vi "3_AdvancedDemo_MHT3.vi"() -> ()   [LabVIEW 2017]
uses:
  Types/MH_InputChannel.ctl
  Types/MH_UIThread_Cmds.ctl
  Types/MH_UIThread_Data.ctl
  _lib/PQ/MultiHarp/MH_InitInfo.ctl
  Types/MH_DataProcThread_QData.ctl
  Types/MH_DataProcThread_QCmds.ctl
  Types/MH_VisThread_QData.ctl
  Types/MH_VisThread_QCmds.ctl
  Types/MH_VisThread_Data.ctl
  _lib/PQ/MultiHarp/MH_RefSource.ctl
  _lib/PQ/MultiHarp/MH_MeasMode.ctl
  <vilib>/Utility/error.llb/DialogType.ctl
  _lib/PQ/MultiHarp/mhlib_x86_x64_UIThread.llb/MH_DllPath_global.vi
  <vilib>/Utility/error.llb/Error Cluster From Error Code.vi
  _lib/PQ/MultiHarp/MH_LibVersion_global.vi
  <vilib>/ErrorRing/Error Ring.xnode
panel:
  in  "Settings":bool=TRUE
  in  "Run continuously":bool caption="Conti."
  in  "Start":bool
  in  "Scale":bool
  out "CountRates":i32[](graph)
  in  "HistoAcqTime":dbl=1.0 caption="Int.Time    s" min=0.1 max=360000.0 step=0.1
  in  "AcqTime":i32=360000000 caption="T3Acq.   ms" min=1 max=360000 step=1
  in  "Binning":i32(ring) caption="Resol.      ps" items=["80", "160", "320", "640", "1280", "2560", "5120", "10240", "20480", "40960", "81920", "163840", "327680", "655360", "1310720", "2621440", "5242880", "10485760", "20971520", "41943040", "83886080", "167772160", "335544320", "671088640", "1342177280", "2684354560"]
  in  "HistoOffset":i32 caption="Offset      ns" min=0 max=100000000 step=1
  out "DeltaT":dbl=3.2767475720388473 caption="Resol.     ms" format="%.2f"
  in  "BitShift":i32=15 min=0 max=32 step=1
  in  "OvlLevel":i32=65536 caption="Ovl.Level" min=1024 max=65536 step=1024
  in  "StopOvl.":bool=TRUE
  out "TTraceGraph":T1(graph)={0.0, "Resolution"=0.0032767475720388473, "Histogram"=[]}
  out "HistoGraph":cluster{dbl, "Resol":dbl, "Histos":u32[][]}(graph)={0.0, "Resol"=0.08, "Histos"=[]}
  in  "SyncEdge":i32(ring) caption="Edge" items=["falling", "rising"]
  in  "SyncDivider":i32(ring)=3 caption="Divider" items=["1", "2", "4", "8", "16"]
  in  "SyncOffset":i32 caption="Offset      ps" min=-99999 max=99999 step=1
  in  "SyncLevel":i32=-50 caption="Level      mV" min=-1200 max=1200 step=1
  in  "Channels":T2[](array[typedef])=[{"Name"="Inp.Chan 1", "Enable"=TRUE, "Offset"=0, "Level"=-50, "Edge"=0}, {"Name"="Inp.Chan 2", "Enable"=TRUE, "Offset"=0, "Level"=-50, "Edge"=0}, {"Name"="Inp.Chan 3", "Enable"=TRUE, "Offset"=0, "Level"=-50, "Edge"=0}, {"Name"="Inp.Chan 4", "Enable"=TRUE, "Offset"=0, "Level"=-50, "Edge"=0}, {"Name"="Inp.Chan 5", "Enable"=TRUE, "Offset"=0, "Level"=-50, "Edge"=0}, {"Name"="Inp.Chan 6", "Enable"=TRUE, "Offset"=0, "Level"=-50, "Edge"=0}, {"Name"="Inp.Chan 7", "Enable"=TRUE, "Offset"=0, "Level"=-50, "Edge"=0}, {"Name"="Inp.Chan 8", "Enable"=TRUE, "Offset"=0, "Level"=-50, "Edge"=0}] {"Edge" items=["falling", "rising"]; "Offset" min=-99999 max=99999 step=80; "Level" min=-1200 max=1200 step=1}
  out "SyncRate":string="Sync Rate: 10000160 cps\n"
  out "OverRun":bool caption="Overrun:"
  out "Status":string="Elements in Q: 0"
  # "Histogram"
  # "Time Trace"
  # "Sync"
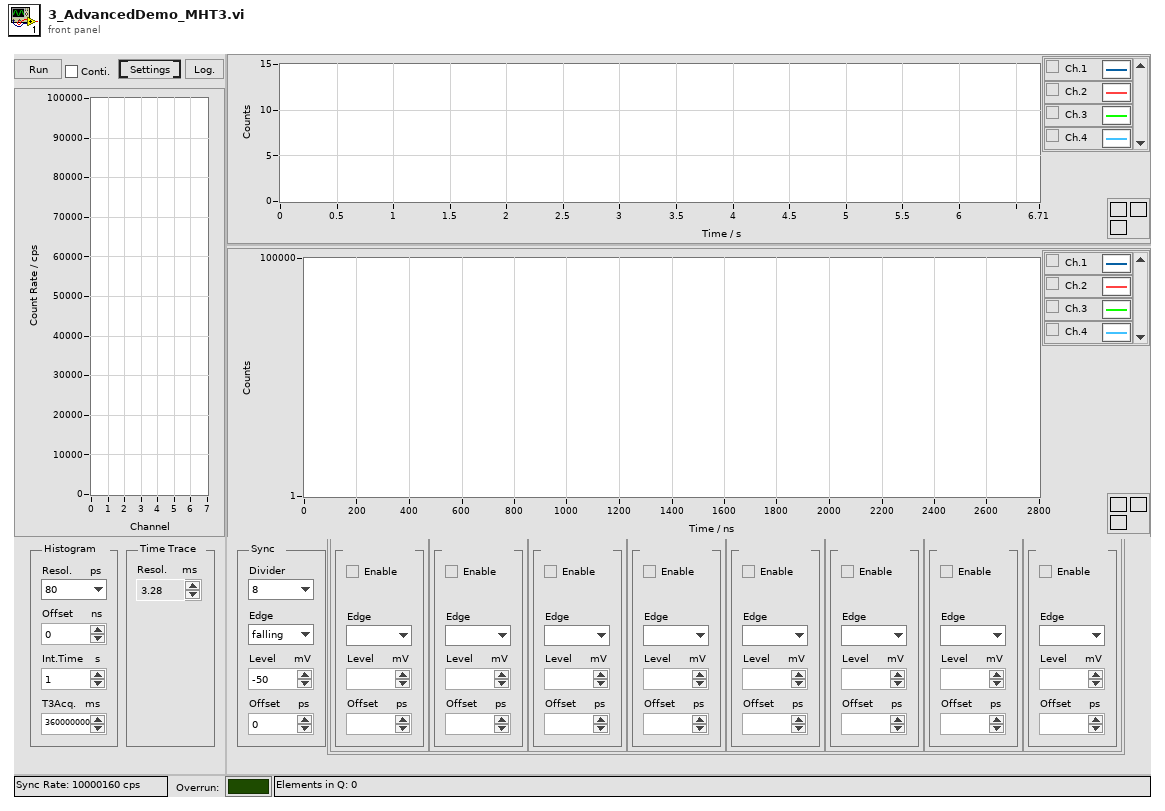
[diagram p1: front panel]
types:
  T1 = cluster{dbl, "Resolution":dbl, "Histogram":u32[][]}
  T2 = typedef "MH_InputChannel.ctl" = cluster{"Name":string, "Enable":bool, "Offset":i32, "Level":i32, "Edge":i32}
  T3 = typedef "MH_DataProcThread_QCmds.ctl" = enum16{"Exit", "Proc", "Init", "SetShift", "SetNumChannels", "SetHistAcqTime"}
  T4 = typedef "MH_VisThread_Data.ctl" = cluster{"Resol":dbl, "DeltaT":dbl, "NumChannels":i32}
  T5 = typedef "MH_VisThread_QData.ctl" = cluster{"Histos":u32[][], "Cmd":T6, "TimeTrace":u32[][], "Bin":i32, "Total bin":u64, "Status":string, "Resol":dbl, "DeltaT":dbl, "nChannels":i32}
  T6 = typedef "MH_VisThread_QCmds.ctl" = enum16{"_none_", "Resol", "nChannels", "DeltaT", "Histo", "TTrace", "Status"}
  T7 = typedef "MH_DataProcThread_QData.ctl" = cluster{"Cmd":T3, "nActual":i32, "Buffer":u32[], "TickCount":u32, "Param":i32}
  T8 = typedef "MH_UIThread_Data.ctl" = cluster{"Init Info":T9, "DevIdx":i32, "SyncDivider":i32, "SyncOffset":i32, "SyncLevel":i32, "Channels":T2[], "CurrentChannels":i32[], "AcqTime":i32, "Binning":i32, "HistoOffset":i32, "HistoLen":i32, "StopOvl.":bool, "OvlLevel":u32, "SyncEdge":i32, "StartMeas":bool, "HistoLength":i32, "Resolution":dbl, "Run cont.":bool, "Status":string, "SyncRate":i32, "BitShift":i32, "HistoAcqTime":dbl}
  T9 = typedef "MH_InitInfo.ctl" = cluster{"Library Version":string, "Serial No.":string, "Model":string, "Partnum":string, "Version":string, "features":i32, "nchannels":i32, "Base Resolution":dbl, "Bin Steps":i32}
  T10 = typedef "MH_UIThread_Cmds.ctl" = enum16{"Idle", "Init", "SetInpChanEnable", "SetInpChanOffset", "SetInpChanTrg", "SetSyncDivider", "SetSyncTrg", "SetSyncOffset", "SetBinning", "SetHistoOffset", "SetHistoLen", "SetStopOvl", "SetBitShift", "SetHistoAcqTime", "GetRates", "GetAllRates", "StartMeas", "StopMeas", "AbortMeas", "GetResolution", "GetHistos", "GetAllHistos", "ReadFiFo", "WriteStatus", "Resize", "EnableControls", "DisableControls", "Error", "Exit"}
  T11 = enum8{"Enabled", "Disabled", "Disabled and Grayed Out"}
  T12 = typedef "MH_MeasMode.ctl" = i32
  T13 = typedef "MH_RefSource.ctl" = enum16{"INTERNAL", "EXTERNAL_10MHZ", "WR_MASTER_GENERIC", "WR_SLAVE_GENERIC", "WR_GRANDM_GENERIC", "EXTN_GPS_PPS", "EXTN_GPS_PPS_UART", "WR_MASTER_MHARP", "WR_SLAVE_MHARP", "WR_GRANDM_MHARP"}
  T14 = typedef "DialogType.ctl" = u16
  T15 = cluster{"T0":dbl, "dt":dbl, "TimeTrace_out":u32[][]}
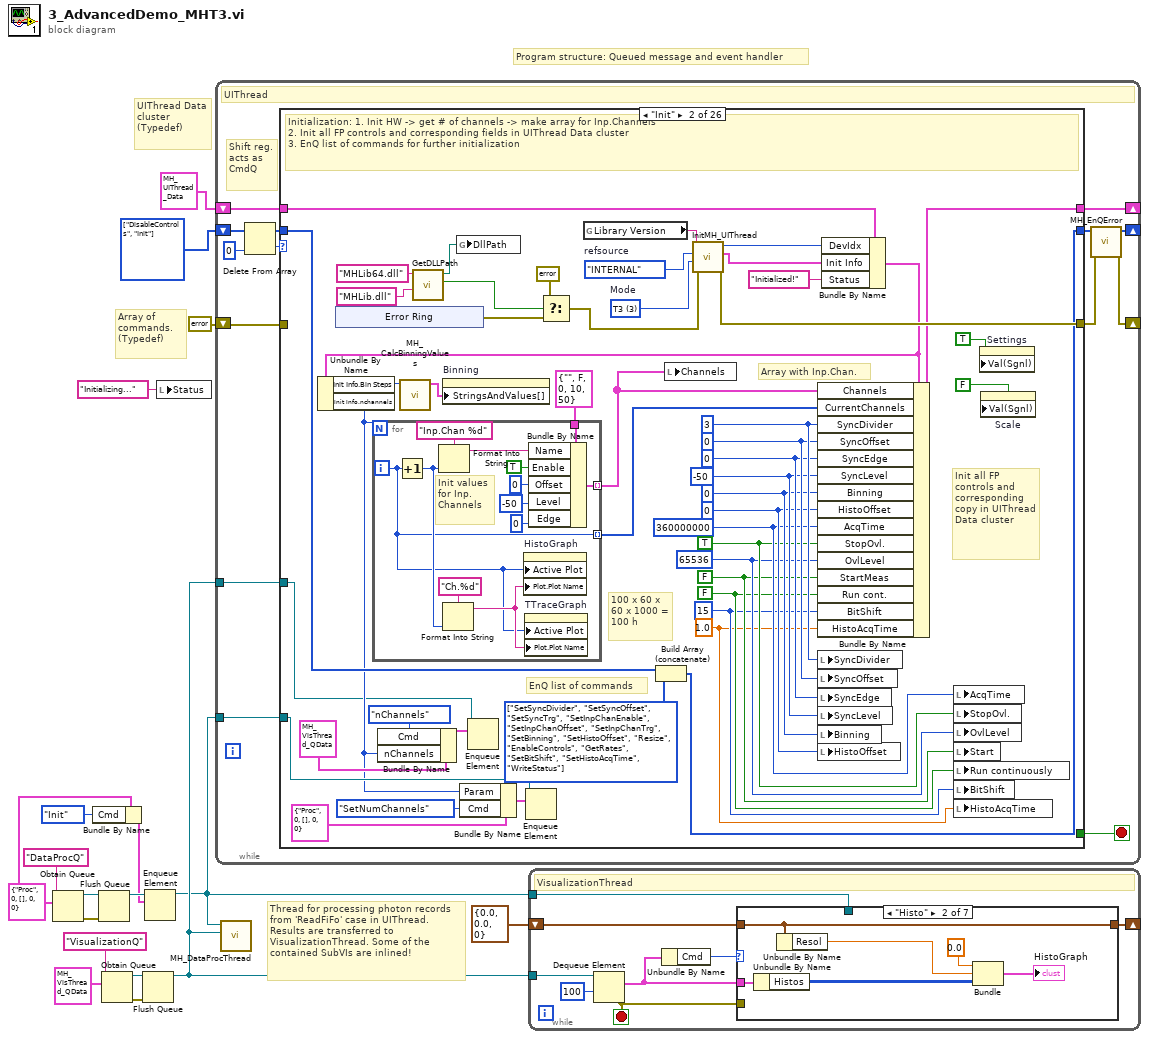
[diagram p0: block diagram]
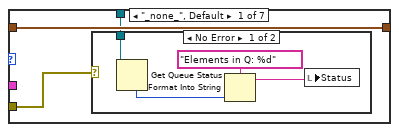
[diagram p2: hidden frame]
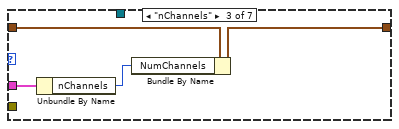
[diagram p4: hidden frame]
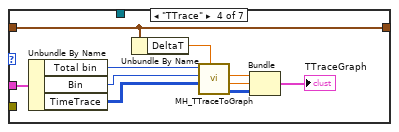
[diagram p5: hidden frame]
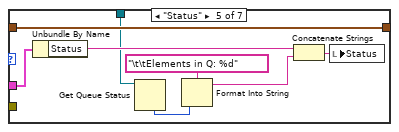
[diagram p6: hidden frame]
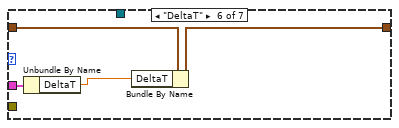
[diagram p7: hidden frame]
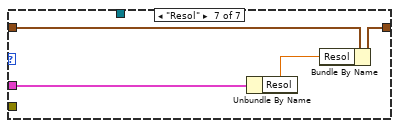
[diagram p8: hidden frame]
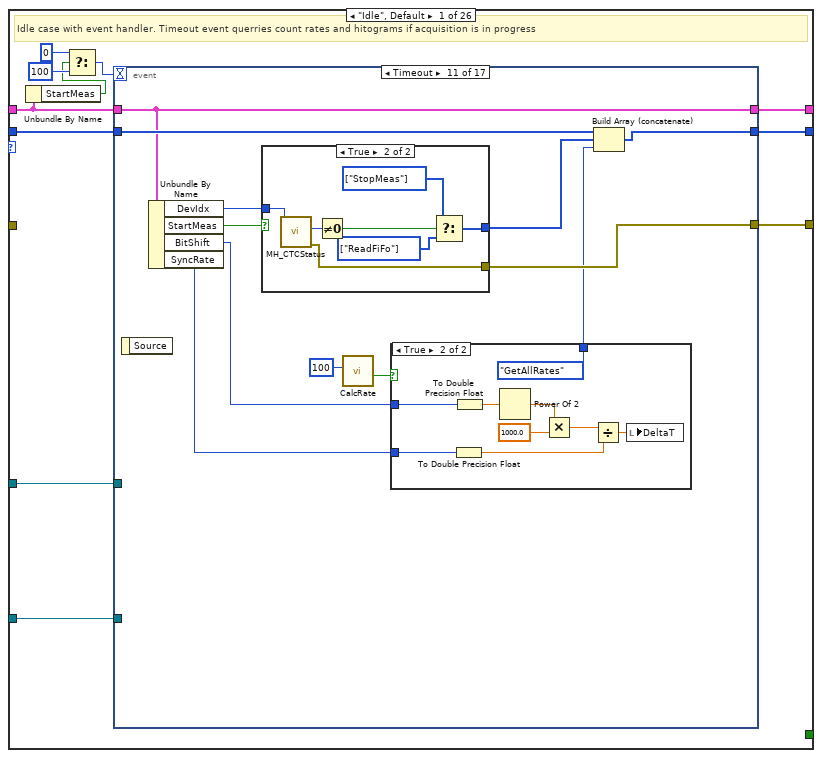
[diagram p9: hidden frame]
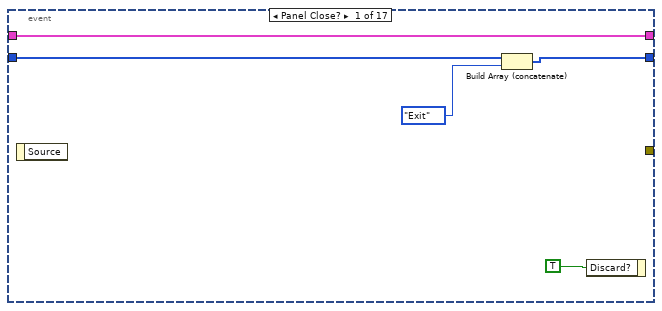
[diagram p10: hidden frame]
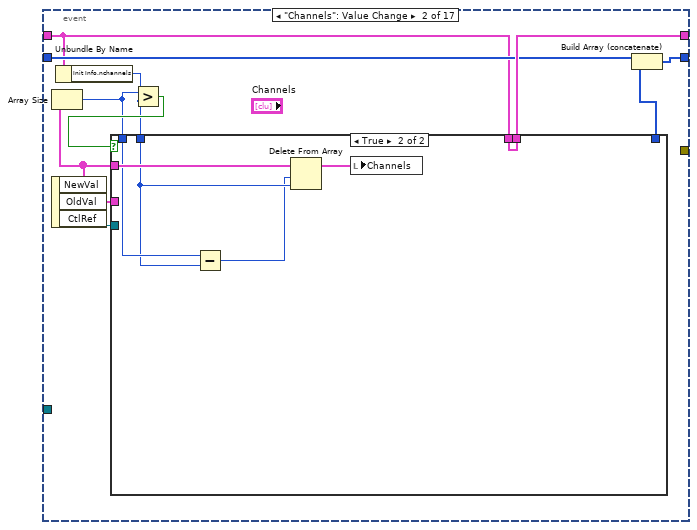
[diagram p11: hidden frame]
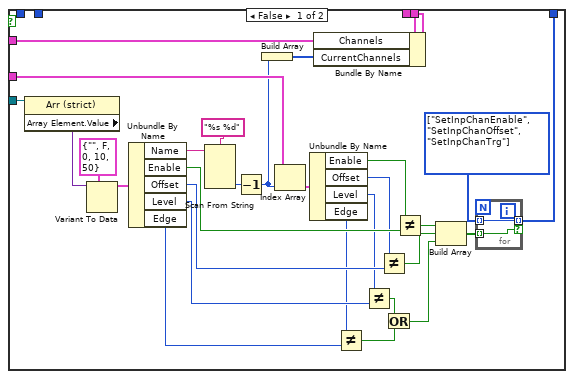
[diagram p12: hidden frame]
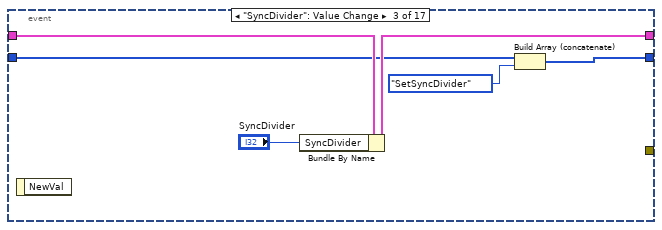
[diagram p13: hidden frame]
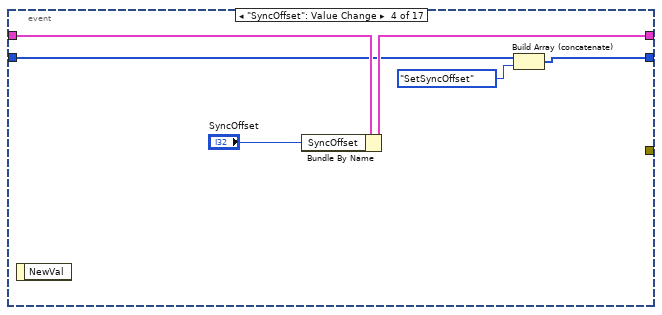
[diagram p14: hidden frame]
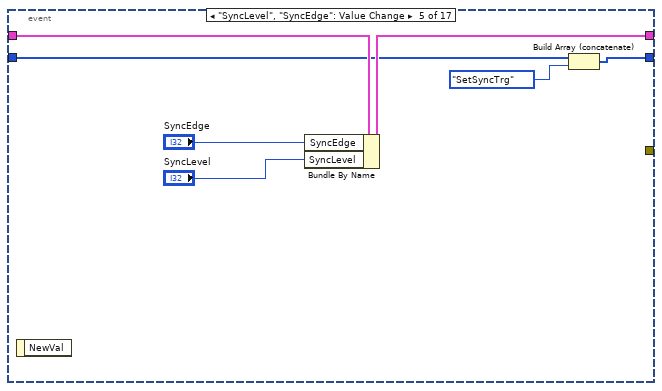
[diagram p15: hidden frame]
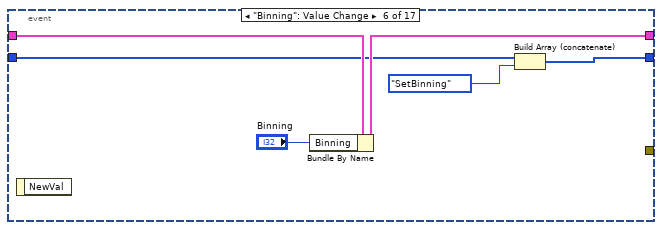
[diagram p16: hidden frame]
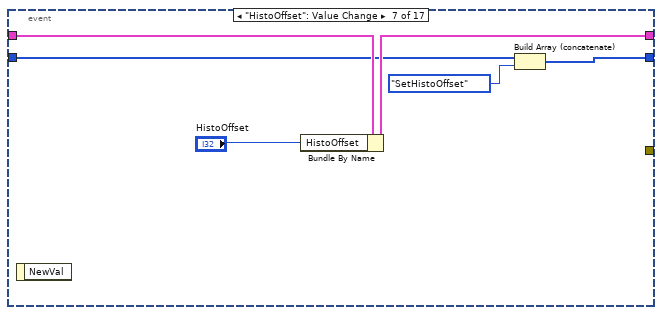
[diagram p17: hidden frame]
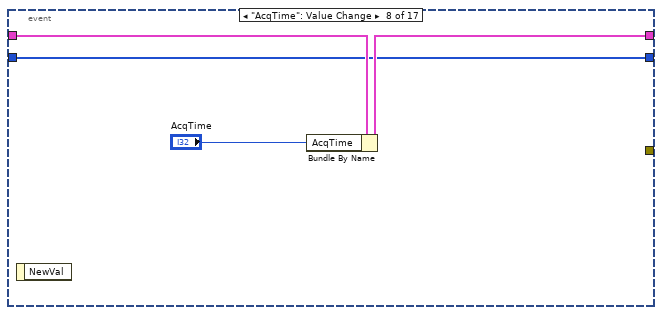
[diagram p18: hidden frame]
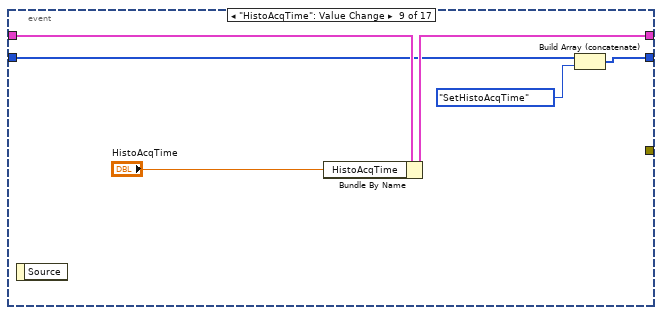
[diagram p19: hidden frame]
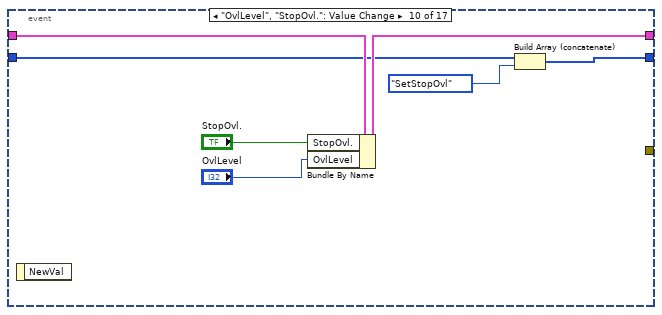
[diagram p20: hidden frame]
diagram:
  w4 = T7 {"Cmd"=enum."Proc", "nActual"=0, "Buffer"=[], "TickCount"=0, "Param"=0} ("MH_DataProcThread_QData")
  w17 = T10[] [enum."DisableControls", enum."Init"] items=["Idle", "Init", "SetInpChanEnable", "SetInpChanOffset", "SetInpChanTrg", "SetSyncDivider", "SetSyncTrg", "SetSyncOffset", "SetBinning", "SetHistoOffset", "SetHistoLen", "SetStopOvl", "SetBitShift", "SetHistoAcqTime", "GetRates", "GetAllRates", "StartMeas", "StopMeas", "AbortMeas", "GetResolution", "GetHistos", "GetAllHistos", "ReadFiFo", "WriteStatus", "Resize", "EnableControls", "DisableControls", "Error", "Exit"]
  # "Thread for processing photon records from 'ReadFiFo' case in UIThread. Results are transferred to VisualizationThread. Some of the contained SubVIs are inlined!"
  # "Array of commands.\n(Typedef)"
  # "Program structure: Queued message and event handler"
  # "UIThread Data cluster\n(Typedef)"
  n1 = Obtain Queue(name (unnamed)="DataProcQ", element data type=w4) -> (queue out=w14:refnum<queue>, error out=w13:errorcluster)  [unwired: 3 in, 1 out]
  n2 = Bundle By Name(cluster=w4, "Cmd"=MH_DataProcThread_QCmds."Init") -> (w2:T7)
  n3 = Flush Queue(queue=w14, error in (no error)=w13) -> (queue out=w5:refnum<queue>)  [unwired: 2 out]
  n4 = Obtain Queue(name (unnamed)="VisualizationQ", element data type=T5 {"Histos"=[], "Cmd"=enum."_none_", "TimeTrace"=[], "Bin"=0, "Total bin"=0, "Status"="", "Resol"=0.0, "DeltaT"=0.0, "nChannels"=0} ("MH_GUIThread_QData")) -> (queue out=w12:refnum<queue>, error out=w11:errorcluster)  [unwired: 3 in, 1 out]
  n5 = Flush Queue(queue=w12, error in (no error)=w11) -> (queue out=w7:refnum<queue>)  [unwired: 2 out]
  n6 = Enqueue Element(queue=w5, element=w2) -> (queue out=w1:refnum<queue>)  [unwired: 2 in, 2 out]
  n7 = local write "Status"("Initializing..." ("Status")) -> ()
  n8 = while {
    shift-right: [w21] -> _
    shift-left: w17 -> [w28]
    shift-right: [w31] -> _
    shift-left: T8 {"Init Info"={"Library Version"="", "Serial No."="", "Model"="", "Partnum"="", "Version"="", "features"=0, "nchannels"=0, "Base Resolution"=0.0, "Bin Steps"=0}, "DevIdx"=0, "SyncDivider"=1, "SyncOffset"=0, "SyncLevel"=50, "Channels"=[], "CurrentChannels"=[], "AcqTime"=1, "Binning"=1, "HistoOffset"=1, "HistoLen"=1024, "StopOvl."=FALSE, "OvlLevel"=1024, "SyncEdge"=10, "StartMeas"=FALSE, "HistoLength"=0, "Resolution"=0.0, "Run cont."=FALSE, "Status"="", "SyncRate"=0, "BitShift"=0, "HistoAcqTime"=0.0} -> [w30]
    shift-right: [w23] -> _
    shift-left: errorcluster {"status"=FALSE, "code"=0, "source"=""} ("error IO") -> [w29]
    tunnel: w1 -> [w20]
    tunnel: w7 -> [w19]
    stop <- w32 stop-if-true
    # "Shift reg.\nacts as\nCmdQ"
    # "UIThread"
    n9 = Delete From Array(array=w28, index=0) -> (deleted portion=w26:T10, array with subset deleted=w25:T10[])  [unwired: 1 in]
    n10 = case shown="\"Init\"" w26 {
      tunnel: [w43 w272 w301 w315 w329 w346 w355 w357 w364 w372 w379 w399 w411 w421 w433 w453 w459 w472 w489 w490 w516 w529 w536 w548 w554 w560] -> w22
      tunnel: [_ _ _ _ _ _ _ _ _ _ _ _ _ _ _ _ _ _ _ _ _ _ _ _ _ TRUE] -> w32
      tunnel: [w42 w253 w304 w318 w332 w348 w356 w361 w368 w373 w380 w384 w401 w415 w425 w457 w462 w474 w485 w500 w515 w517 w535 w547 w555 w563] -> w31
      tunnel: w30 -> [w39 w258 w304 w318 w332 w348 w356 w361 w368 w373 w380 w384 w401 w415 w426 w457 w463 w475 w486 w500 w515 w517 w535 w547 w555 w563]
      tunnel: [w40 w277 w302 w316 w330 w344 w354 w360 w367 w371 w378 _ _ w414 w432 w456 w465 w477 w487 w495 _ _ _ _ _ w561] -> w24
      tunnel: w29 -> [_ _ _ _ _ _ _ _ _ _ _ _ _ _ _ _ _ _ _ _ _ _ _ _ w556 _]
      tunnel: w25 -> [w41 w274 w301 w315 w329 w346 w355 w357 w363 w372 w379 w399 w411 w421 w433 w454 w460 w472 w489 w491 w516 w529 w536 w548 _ w560]
      tunnel: w20 -> [w34 w251 _ _ _ _ _ _ _ _ _ w385 w402 _ _ w450 _ _ _ w492 _ _ _ _ _ w559]
      tunnel: w19 -> [w33 w243 _ _ _ _ _ _ _ _ _ w386 _ _ _ _ _ _ w482 _ _ _ _ _ _ w558]
      frame "Idle", Default {
        # "Idle case with event handler. Timeout event querries count rates and hitograms if acquisition is in progress"
        n11 = Unbundle By Name(w39) -> ("StartMeas"=w37:bool)
        n12 = Select(t=0, s=w37, f=100) -> (s? t:f=w36:i32)
        n13 = event shown="[10] Timeout" {
          selector: _ -> [_ _ _ _ _ _ _ _ _ _ _ _ _ _ _ _ _]
          dyn-events: _ -> [_ _ _ _ _ _ _ _ _ _ _ _ _ _ _ _ _]
          timeout: w36 -> [_ _ _ _ _ _ _ _ _ _ _ _ _ _ _ _ _]
          tunnel: [w44 w54 w98 w104 w111 w118 w124 w129 w134 w141 w156 w174 w186 w204 w210 w218 w228] -> w43
          tunnel: [w47 w57 w102 w108 w115 w121 w127 w131 w137 w144 w155 w178 w185 w202 w209 w217 w231] -> w42
          tunnel: w39 -> [w47 w53 w103 w109 w116 w122 w128 w132 w138 w145 w155 w179 w183 w203 w209 w217 w231]
          tunnel: w41 -> [w46 w56 w100 w106 w113 w120 w126 w129 w135 w143 w157 w175 w187 w204 w210 w218 w229]
          tunnel: [_ _ _ _ _ _ _ _ _ _ w151 _ _ _ _ _ _] -> w40
          tunnel: w34 -> [_ _ _ _ _ _ _ _ _ _ _ _ _ _ _ _ _]
          tunnel: w33 -> [_ _ _ _ _ _ _ _ _ _ _ _ _ _ _ _ _]
          event Panel Close? {
            n14 = event-data() -> ()  [unwired: 1 in, 1 out]
            n15 = Build Array (concatenate)(w46, MH_UIThread_Cmds."Exit") -> (w44:T10[])
            n16 = event-data("Discard?"=TRUE) -> ()  [unwired: 1 in, 1 out]
          }
          event "Channels": Value Change {
            n17 = event-data() -> ("NewVal"=w52:T2[], "OldVal"=w58:T2[], "CtlRef"=w59:refnum<vi>)  [unwired: 1 in]
            n18 = Array Size(array=w52) -> (size(s)=w49:i32)
            n19 = Unbundle By Name(w53) -> ("Init Info.nchannels"=w50:i32)
            n20 = Greater?(x=w49, y=w50) -> (0:w51:bool)
            n21 = case shown="True" w51 {
              tunnel: w59 -> [w89 _]
              tunnel: w58 -> [w83 _]
              tunnel: [w66 w97] -> w57
              tunnel: [w64 _] -> w55
              tunnel: w53 -> [w61 w97]
              tunnel: w52 -> [w60 w96]
              tunnel: w50 -> [_ w94]
              tunnel: w49 -> [_ w95]
              frame False {
                w67 = T10[] [enum."SetInpChanEnable", enum."SetInpChanOffset", enum."SetInpChanTrg"] items=["Idle", "Init", "SetInpChanEnable", "SetInpChanOffset", "SetInpChanTrg", "SetSyncDivider", "SetSyncTrg", "SetSyncOffset", "SetBinning", "SetHistoOffset", "SetHistoLen", "SetStopOvl", "SetBitShift", "SetHistoAcqTime", "GetRates", "GetAllRates", "StartMeas", "StopMeas", "AbortMeas", "GetResolution", "GetHistos", "GetAllHistos", "ReadFiFo", "WriteStatus", "Resize", "EnableControls", "DisableControls", "Error", "Exit"]
                n22 = property class="Arr (strict)"(reference=w89) -> ("Array Element.Value"=w88:variant)  [unwired: 1 in, 2 out]
                n23 = Variant To Data(type=T2 {"Name"="", "Enable"=FALSE, "Offset"=0, "Level"=10, "Edge"=50} ("Channel"), Variant=w88) -> (data=w65:T2)  [unwired: 1 in, 1 out]
                n24 = Unbundle By Name(w65) -> ("Name"=w86:string, "Enable"=w80:bool, "Offset"=w78:i32, "Level"=w76:i32, "Edge"=w74:i32)
                n25 = Scan From String(format string="%s %d", input string=w86) -> (output 2=w84:i32)  [unwired: 5 in, 3 out]
                n26 = Decrement(x=w84) -> (x-1=w63:i32)
                n27 = Build Array(w63) -> (w62:i32[])
                n28 = Index Array(array=w83, index=w63) -> (element=w82:T2)
                n29 = Unbundle By Name(w82) -> ("Enable"=w81:bool, "Offset"=w79:i32, "Level"=w77:i32, "Edge"=w75:i32)
                n30 = Bundle By Name(cluster=w61, "Channels"=w60, "CurrentChannels"=w62) -> (w66:T8)
                n31 = Not Equal?(x=w75, y=w74) -> (x != y?=w69:bool)
                n32 = Not Equal?(x=w77, y=w76) -> (x != y?=w70:bool)
                n33 = Not Equal?(x=w79, y=w78) -> (x != y?=w72:bool)
                n34 = Or(x=w70, y=w69) -> (x .or. y?=w68:bool)
                n35 = Not Equal?(x=w81, y=w80) -> (x != y?=w73:bool)
                n36 = Build Array(w73, w72, w68) -> (w71:bool[])
                n37 = for {
                  tunnel: w71 -> [w90] mode=indexing
                  tunnel: w67 -> [w91] mode=indexing
                  tunnel: [w91] -> w64 mode=indexing if=w90
                }
              }
              frame True {
                n38 = Subtract(x=w95, y=w94) -> (x-y=w93:i32)
                n39 = Delete From Array(array=w96, length=w93, index=w94) -> (array with subset deleted=w92:T2[])  [unwired: 1 out]
                n40 = local write "Channels"(w92) -> ()
              }
            }
            n41 = Build Array (concatenate)(w56, w55) -> (w54:T10[])
          }
          event "SyncDivider": Value Change {
            n42 = event-data() -> ()  [unwired: 1 in, 1 out]
            n43 = Bundle By Name(cluster=w103, "SyncDivider"="SyncDivider") -> (w102:T8)
            n44 = Build Array (concatenate)(w100, MH_UIThread_Cmds."SetSyncDivider") -> (w98:T10[])
          }
          event "SyncOffset": Value Change {
            n45 = event-data() -> ()  [unwired: 1 in, 1 out]
            n46 = Bundle By Name(cluster=w109, "SyncOffset"="SyncOffset") -> (w108:T8)
            n47 = Build Array (concatenate)(w106, MH_UIThread_Cmds."SetSyncOffset") -> (w104:T10[])
          }
          event "SyncLevel", "SyncEdge": Value Change {
            n48 = event-data() -> ()  [unwired: 1 in, 1 out]
            n49 = Bundle By Name(cluster=w116, "SyncEdge"="SyncEdge", "SyncLevel"="SyncLevel") -> (w115:T8)
            n50 = Build Array (concatenate)(w113, MH_UIThread_Cmds."SetSyncTrg") -> (w111:T10[])
          }
          event "Binning": Value Change {
            n51 = event-data() -> ()  [unwired: 1 in, 1 out]
            n52 = Bundle By Name(cluster=w122, "Binning"="Binning") -> (w121:T8)
            n53 = Build Array (concatenate)(w120, MH_UIThread_Cmds."SetBinning") -> (w118:T10[])
          }
          event "HistoOffset": Value Change {
            n54 = event-data() -> ()  [unwired: 1 in, 1 out]
            n55 = Bundle By Name(cluster=w128, "HistoOffset"="HistoOffset") -> (w127:T8)
            n56 = Build Array (concatenate)(w126, MH_UIThread_Cmds."SetHistoOffset") -> (w124:T10[])
          }
          event "AcqTime": Value Change {
            n57 = event-data() -> ()  [unwired: 1 in, 1 out]
            n58 = Bundle By Name(cluster=w132, "AcqTime"="AcqTime") -> (w131:T8)
          }
          event "HistoAcqTime": Value Change {
            n59 = event-data() -> ()  [unwired: 1 in, 1 out]
            n60 = Bundle By Name(cluster=w138, "HistoAcqTime"="HistoAcqTime") -> (w137:T8)
            n61 = Build Array (concatenate)(w135, MH_UIThread_Cmds."SetHistoAcqTime") -> (w134:T10[])
          }
          event "OvlLevel", "StopOvl.": Value Change {
            n62 = event-data() -> ()  [unwired: 1 in, 1 out]
            n63 = Bundle By Name(cluster=w145, "StopOvl."="StopOvl.", "OvlLevel"="OvlLevel") -> (w144:T8)
            n64 = Build Array (concatenate)(w143, MH_UIThread_Cmds."SetStopOvl") -> (w141:T10[])
          }
          event Timeout {
            n65 = event-data() -> ()  [unwired: 1 in, 1 out]
            n66 = Unbundle By Name(w155) -> ("DevIdx"=w153:i32, "StartMeas"=w154:bool, "BitShift"=w150:i32, "SyncRate"=w149:i32)
            n67 = case shown="True" w154 {
              tunnel: w153 -> [_ w173]
              tunnel: [_ w171] -> w152
              tunnel: [_ w168] -> w151
              frame False {
              }
              frame True {
                w169 = T10[] [enum."ReadFiFo"] items=["Idle", "Init", "SetInpChanEnable", "SetInpChanOffset", "SetInpChanTrg", "SetSyncDivider", "SetSyncTrg", "SetSyncOffset", "SetBinning", "SetHistoOffset", "SetHistoLen", "SetStopOvl", "SetBitShift", "SetHistoAcqTime", "GetRates", "GetAllRates", "StartMeas", "StopMeas", "AbortMeas", "GetResolution", "GetHistos", "GetAllHistos", "ReadFiFo", "WriteStatus", "Resize", "EnableControls", "DisableControls", "Error", "Exit"]
                w170 = T10[] [enum."StopMeas"] items=["Idle", "Init", "SetInpChanEnable", "SetInpChanOffset", "SetInpChanTrg", "SetSyncDivider", "SetSyncTrg", "SetSyncOffset", "SetBinning", "SetHistoOffset", "SetHistoLen", "SetStopOvl", "SetBitShift", "SetHistoAcqTime", "GetRates", "GetAllRates", "StartMeas", "StopMeas", "AbortMeas", "GetResolution", "GetHistos", "GetAllHistos", "ReadFiFo", "WriteStatus", "Resize", "EnableControls", "DisableControls", "Error", "Exit"]
                n68 = call "MH_CTCStatus.vi"("devidx"=w173) -> ("error out"=w168:errorcluster, "ctcstatus"=w172:i32)  [unwired: 8 in, 1 out]
                n69 = Not Equal To 0?(x=w172) -> (x != 0?=w167:bool)
                n70 = Select(t=w170, s=w167, f=w169) -> (s? t:f=w171:T10[])
              }
            }
            n71 = call "CalcRate.vi"("Refresh(ms)"=u32 100) -> ("updated?"=w147:bool)  [unwired: 8 in, 2 out]
            n72 = case shown="True" w147 {
              tunnel: w150 -> [_ w160]
              tunnel: w149 -> [_ w159]
              tunnel: [_ MH_UIThread_Cmds."GetAllRates"] -> w148
              frame False {
              }
              frame True {
                n73 = To Double Precision Float(number=w159) -> (double precision float=w164:dbl)
                n74 = To Double Precision Float(number=w160) -> (double precision float=w165:dbl)
                n75 = Power Of 2(x=w165) -> (2^x=w163:dbl)
                n76 = Multiply(x=w163, y=1000.0) -> (x*y=w162:dbl)
                n77 = Divide(x=w162, y=w164) -> (x/y=w166:dbl)
                n78 = local write "DeltaT"(w166) -> ()
              }
            }
            n79 = Build Array (concatenate)(w157, w152, w148) -> (w156:T10[])
          }
          event "BitShift": Value Change {
            n80 = event-data() -> ()  [unwired: 1 in, 1 out]
            n81 = Bundle By Name(cluster=w179, "BitShift"="BitShift") -> (w178:T8)
            n82 = Build Array (concatenate)(w175, MH_UIThread_Cmds."SetBitShift") -> (w174:T10[])
          }
          event "Start": Value Change {
            n83 = event-data() -> ()  [unwired: 1 in, 1 out]
            n84 = Unbundle By Name(w183) -> ("SyncRate"=w182:i32)
            n85 = Greater Or Equal?(x=w182, y=10) -> (x >= y?=w180:bool)
            n86 = case shown="True" w180 {
              selector: w180 -> [w189 _]
              tunnel: w187 -> [w191 w200]
              tunnel: [w191 w198] -> w186
              tunnel: [w190 w197] -> w185
              tunnel: "Start" -> [_ w196]
              tunnel: w183 -> [w190 w192]
              frame False {
                n87 = local write "Start"(w189) -> ()
                n88 = One Button Dialog(message="SyncRate too low!!!" ("Status")) -> ()  [unwired: 1 in, 1 out]
              }
              frame True {
                w195 = T10[] [enum."SetBitShift", enum."SetHistoAcqTime", enum."StartMeas"] items=["Idle", "Init", "SetInpChanEnable", "SetInpChanOffset", "SetInpChanTrg", "SetSyncDivider", "SetSyncTrg", "SetSyncOffset", "SetBinning", "SetHistoOffset", "SetHistoLen", "SetStopOvl", "SetBitShift", "SetHistoAcqTime", "GetRates", "GetAllRates", "StartMeas", "StopMeas", "AbortMeas", "GetResolution", "GetHistos", "GetAllHistos", "ReadFiFo", "WriteStatus", "Resize", "EnableControls", "DisableControls", "Error", "Exit"]
                n89 = Bundle By Name(cluster=w192, "StartMeas"=w196) -> (w197:T8)
                n90 = Build Array(MH_UIThread_Cmds."AbortMeas") -> (w193:T10[])
                n91 = Select(t=w195, s=w196, f=w193) -> (s? t:f=w199:T10[])
                n92 = Build Array (concatenate)(w200, w199) -> (w198:T10[])
              }
            }
          }
          event "Run continuously": Value Change {
            n93 = event-data() -> ()  [unwired: 1 in, 1 out]
            n94 = Bundle By Name(cluster=w203, "Run cont."="Run continuously") -> (w202:T8)
          }
          event "Scale": Value Change {
            n95 = event-data() -> ()  [unwired: 1 in, 1 out]
            n96 = Select(t=u8 0 ("Y Scale.Mapping Mode"), s="Scale", f=u8 1 ("Y Scale.Mapping Mode")) -> (s? t:f=w205:u8)
            n97 = property on="HistoGraph" class="WFGraph (strict)"("YScale.Mapping Mode"=w205) -> ()  [unwired: 2 in, 2 out]
          }
          event "Settings": Value Change {
            n98 = event-data() -> ()  [unwired: 1 in, 1 out]
            n99 = property on="Splitter" class="Splitter"() -> ("Position"=w216:i32)  [unwired: 2 in, 2 out]
            n100 = Select(t=237 ("PosT"), s="Settings", f=0 ("PosF")) -> (s? t:f=w213:i32)
            n101 = Subtract(x=w216, y=w213) -> (x-y=w212:i32)
            n102 = while {
              shift-right: [w227] -> _
              shift-left: w212 -> [w220]
              i -> [w226]
              stop <- w223 stop-if-true
              n103 = property on="Splitter 4" class="Splitter"("Position"=w220) -> (error out=w219:errorcluster)  [unwired: 2 in, 1 out]
              n104 = Greater Or Equal?(x=w226, y=10) -> (x >= y?=w224:bool)
              n105 = Decrement(x=w220) -> (x-1=w227:i32)
              n106 = Unbundle(w219) -> ("status"=w222:bool)  [unwired: 2 out]
              n107 = Not(x=w222) -> (.not. x?=w221:bool)
              n108 = Or(x=w221, y=w224) -> (x .or. y?=w223:bool)
            }
          }
          event Panel Resize {
            n109 = event-data() -> ()  [unwired: 1 in, 1 out]
            n110 = Build Array (concatenate)(w229, MH_UIThread_Cmds."Resize") -> (w228:T10[])
          }
        }
      }
      frame "Init" {
        w232 = T12 3 items=["HIST"=0, "T2"=2, "T3"=3]  # Mode
        w234 = MH_RefSource."INTERNAL"  # refsource
        w241 = 1.0 ("HistoAcqTime")
        w242 = 15 ("Value (Signaling)")
        w260 = FALSE ("Run cont.")
        w262 = FALSE ("StartMeas")
        w263 = 65536 ("OvlLevel")
        w264 = TRUE ("StopOvl.")
        w265 = 360000000 ("AcqTime")
        w266 = 0 ("HistoOffset")
        w267 = 0 ("Binning")
        w268 = -50 ("SyncLevel")
        w269 = 0 ("SyncZeroX")
        w270 = 0 ("SyncOffset")
        w271 = 3 ("SyncDivider")
        w273 = T10[] [enum."SetSyncDivider", enum."SetSyncOffset", enum."SetSyncTrg", enum."SetInpChanEnable", enum."SetInpChanOffset", enum."SetInpChanTrg", enum."SetBinning", enum."SetHistoOffset", enum."Resize", enum."EnableControls", enum."GetRates", enum."SetBitShift", enum."SetHistoAcqTime", enum."WriteStatus"] items=["Idle", "Init", "SetInpChanEnable", "SetInpChanOffset", "SetInpChanTrg", "SetSyncDivider", "SetSyncTrg", "SetSyncOffset", "SetBinning", "SetHistoOffset", "SetHistoLen", "SetStopOvl", "SetBitShift", "SetHistoAcqTime", "GetRates", "GetAllRates", "StartMeas", "StopMeas", "AbortMeas", "GetResolution", "GetHistos", "GetAllHistos", "ReadFiFo", "WriteStatus", "Resize", "EnableControls", "DisableControls", "Error", "Exit"]
        # "100 x 60 x 60 x 1000 = 100 h"
        # "Init all FP controls and corresponding copy in UIThread Data cluster"
        # "EnQ list of commands"
        # "Array with Inp.Chan."
        # "Initialization: 1. Init HW -> get # of channels -> make array for Inp.Channels\n2. Init all FP controls and corresponding fields in UIThread Data cluster\n3. EnQ list of commands for further initialization"
        n111 = xnode "Error Ring"() -> ("error out"=w235:errorcluster)
        n112 = call "GetDLLPath.vi"("DllName_32bit"="MHLib.dll" ("name or relative path"), "DllName_64bit"="MHLib64.dll" ("name or relative path")) -> ("file exists?"=w237:bool, "DLLPath"=w238:path)  [unwired: 8 in]
        n113 = global write "MH_DllPath_global.vi" "DllPath"(w238) -> ()
        n114 = Select(t=errorcluster {"status"=FALSE, "code"=0, "source"=""} ("error IO"), s=w237, f=w235) -> (s? t:f=w254:errorcluster)
        n115 = global read "MH_LibVersion_global.vi" "Library Version"() -> (w233:string)
        n116 = Build Array (concatenate)(w274, w273) -> (w272:T10[])
        n117 = call "InitMH_UIThread.vi"("error in (no error)"=w254, "Mode"=w232, "refsource"=w234, "Library Version"=w233) -> ("error out"=w277:errorcluster, "Init Info"=w280:T9, "DevIdx"=w279:i32)  [unwired: 5 in]
        n118 = local write "SyncDivider"(w271) -> ()
        n119 = local write "SyncOffset"(w270) -> ()
        n120 = local write "SyncEdge"(w269) -> ()
        n121 = local write "SyncLevel"(w268) -> ()
        n122 = local write "Binning"(w267) -> ()
        n123 = local write "HistoOffset"(w266) -> ()
        n124 = Bundle By Name(cluster=w258, "DevIdx"=w279, "Init Info"=w280, "Status"="Initialized!") -> (w257:T8)
        n125 = Unbundle By Name(w257) -> ("Init Info.Bin Steps"=w256:i32, "Init Info.nchannels"=w244:i32)
        n126 = for {
          N: w244 -> [_]
          tunnel: T2 {"Name"="", "Enable"=FALSE, "Offset"=0, "Level"=10, "Edge"=50} ("Channel") -> [w297]
          tunnel: [w296] -> w276 mode=indexing
          tunnel: [w286] -> w275 mode=indexing
          i -> [w286]
          # "Init values for Inp. Channels"
          n127 = Increment(x=w286) -> (x+1=w289:i32)
          n128 = Format Into String(format string="Inp.Chan %d", w289) -> (resulting string=w294:string)  [unwired: 2 in, 1 out]
          n129 = Format Into String(format string="Ch.%d", w289) -> (resulting string=w287:string)  [unwired: 2 in, 1 out]
          n130 = property on="HistoGraph" class="WFGraph (strict)"("Active Plot"=w286, "Plot.Plot Name"=w287) -> ()  [unwired: 2 in, 2 out]
          n131 = property on="TTraceGraph" class="WFGraph (strict)"("Active Plot"=w286, "Plot.Plot Name"=w287) -> ()  [unwired: 2 in, 2 out]
          n132 = Bundle By Name(cluster=w297, "Name"=w294, "Enable"=TRUE, "Offset"=0, "Level"=-50 ("CFDZeroX"), "Edge"=0 ("CFDLevel")) -> (w296:T2)
        }
        n133 = Bundle By Name(cluster=T5 {"Histos"=[], "Cmd"=enum."_none_", "TimeTrace"=[], "Bin"=0, "Total bin"=0, "Status"="", "Resol"=0.0, "DeltaT"=0.0, "nChannels"=0} ("MH_GUIThread_QData"), "Cmd"=MH_VisThread_QCmds."nChannels", "nChannels"=w244) -> (w246:T5)
        n134 = call "MH_CalcBinningValues.vi"("Bin Steps"=w256) -> ("BinningValues"=w261:cluster{"String":string, "Value":i32}[])  [unwired: 10 in]
        n135 = property on="Binning" class="Ring (strict)"("StringsAndValues[]"=w261) -> ()  [unwired: 2 in, 2 out]
        n136 = Bundle By Name(cluster=T7 {"Cmd"=enum."Proc", "nActual"=0, "Buffer"=[], "TickCount"=0, "Param"=0} ("MH_DataProcThread_QData"), "Param"=w244, "Cmd"=MH_DataProcThread_QCmds."SetNumChannels") -> (w250:T7)
        n137 = Enqueue Element(queue=w243, element=w246) -> ()  [unwired: 2 in, 3 out]
        n138 = Enqueue Element(queue=w251, element=w250) -> ()  [unwired: 2 in, 3 out]
        n139 = local write "Channels"(w276) -> ()
        n140 = Bundle By Name(cluster=w257, "Channels"=w276, "CurrentChannels"=w275, "SyncDivider"=w271, "SyncOffset"=w270, "SyncEdge"=w269, "SyncLevel"=w268, "Binning"=w267, "HistoOffset"=w266, "AcqTime"=w265, "StopOvl."=w264, "OvlLevel"=w263, "StartMeas"=w262, "Run cont."=w260, "BitShift"=w242, "HistoAcqTime"=w241) -> (w253:T8)
        n141 = local write "AcqTime"(w265) -> ()
        n142 = local write "StopOvl."(w264) -> ()
        n143 = local write "OvlLevel"(w263) -> ()
        n144 = local write "Start"(w262) -> ()
        n145 = local write "Run continuously"(w260) -> ()
        n146 = local write "BitShift"(w242) -> ()
        n147 = local write "HistoAcqTime"(w241) -> ()
        n148 = property on="Settings" class="Bool (strict)"("Val(Sgnl)"=TRUE ("Value (Signaling)")) -> ()  [unwired: 2 in, 2 out]
        n149 = property on="Scale" class="Bool (strict)"("Val(Sgnl)"=FALSE ("Value (Signaling)")) -> ()  [unwired: 2 in, 2 out]
      }
      frame "SetInpChanEnable" {
        n150 = Unbundle By Name(w304) -> ("DevIdx"=w303:i32, "Channels"=w298:T2[], "CurrentChannels"=w299:i32[])
        n151 = for {
          tunnel: w303 -> [w311]
          shift-right: [w310] -> w302
          shift-left: errorcluster {"status"=FALSE, "code"=0, "source"=""} ("error out") -> [w309]
          tunnel: w299 -> [w305] mode=indexing
          tunnel: w298 -> [w308]
          n152 = Index Array(array=w308, index=w305) -> (element=w307:T2)
          n153 = Unbundle By Name(w307) -> ("Enable"=w306:bool)
          n154 = call "MH_SetInputChannelEnable.vi"("error in (no error)"=w309, "enable"=w306, "channel"=w305, "devidx"=w311) -> ("error out"=w310:errorcluster)  [unwired: 6 in, 1 out]
        }
      }
      frame "SetInpChanOffset" {
        n155 = Unbundle By Name(w318) -> ("DevIdx"=w317:i32, "Channels"=w312:T2[], "CurrentChannels"=w313:i32[])
        n156 = for {
          tunnel: w317 -> [w323]
          shift-right: [w320] -> w316
          shift-left: errorcluster {"status"=FALSE, "code"=0, "source"=""} ("error out") -> [w321]
          tunnel: w313 -> [w322] mode=indexing
          tunnel: w312 -> [w325]
          n157 = Index Array(array=w325, index=w322) -> (element=w324:T2)
          n158 = Unbundle By Name(w324) -> ("Offset"=w319:i32)
          n159 = call "MH_SetInputChannelOffset.vi"("error in (no error)"=w321, "Offset"=w319, "channel"=w322, "devidx"=w323) -> ("error out"=w320:errorcluster)  [unwired: 6 in, 1 out]
        }
      }
      frame "SetInpChanTrg" {
        n160 = Unbundle By Name(w332) -> ("DevIdx"=w331:i32, "Channels"=w326:T2[], "CurrentChannels"=w327:i32[])
        n161 = for {
          tunnel: w331 -> [w335]
          shift-right: [w337] -> w330
          shift-left: errorcluster {"status"=FALSE, "code"=0, "source"=""} ("error out") -> [w338]
          tunnel: w327 -> [w336] mode=indexing
          tunnel: w326 -> [w340]
          n162 = Index Array(array=w340, index=w336) -> (element=w339:T2)
          n163 = Unbundle By Name(w339) -> ("Level"=w334:i32, "Edge"=w333:i32)
          n164 = call "MH_SetInputEdgeTrg.vi"("channel"=w336, "error in (no error)"=w338, "edge"=w333, "level"=w334, "devidx"=w335) -> ("error out"=w337:errorcluster)  [unwired: 5 in, 1 out]
        }
      }
      frame "SetSyncDivider" {
        n165 = Unbundle By Name(w348) -> ("DevIdx"=w347:i32, "SyncDivider"=w343:i32)
        n166 = Power Of 2(x=w343) -> (2^x=w342:dbl)
        n167 = To Long Integer(number=w342) -> (32bit integer=w341:i32)
        n168 = call "MH_SetSyncDiv.vi"("SyncDivider"=w341, "devidx"=w347) -> ("error out"=w345:errorcluster)  [unwired: 8 in, 1 out]
        n169 = flat-sequence {
          tunnel: w345 -> [w349]
          tunnel: [w349] -> w344
          frame #0 {
            n170 = Wait (ms)(milliseconds to wait=u32 100) -> ()  [unwired: 1 out]
          }
        }
      }
      frame "SetSyncTrg" {
        n171 = Unbundle By Name(w356) -> ("DevIdx"=w353:i32, "SyncLevel"=w351:i32, "SyncEdge"=w352:i32)
        n172 = call "MH_SetSyncEdgeTrg.vi"("edge"=w352, "level"=w351, "devidx"=w353) -> ("error out"=w354:errorcluster)  [unwired: 7 in, 1 out]
      }
      frame "SetSyncOffset" {
        n173 = Unbundle By Name(w361) -> ("DevIdx"=w359:i32, "SyncOffset"=w358:i32)
        n174 = call "MH_SetSyncChannelOffset.vi"("Offset"=w358, "devidx"=w359) -> ("error out"=w360:errorcluster)  [unwired: 8 in, 1 out]
      }
      frame "SetBinning" {
        # "When binning is changed the new resolution is querried"
        n175 = Unbundle By Name(w368) -> ("DevIdx"=w366:i32, "Binning"=w365:i32)
        n176 = call "MH_SetBinning.vi"("Binning"=w365, "devidx"=w366) -> ("error out"=w367:errorcluster)  [unwired: 8 in, 1 out]
        n177 = Build Array (concatenate)(MH_UIThread_Cmds."GetResolution", w363) -> (w364:T10[])
      }
      frame "SetHistoOffset" {
        n178 = Unbundle By Name(w373) -> ("DevIdx"=w370:i32, "HistoOffset"=w369:i32)
        n179 = call "MH_SetOffset.vi"("Offset"=w369, "devidx"=w370) -> ("error out"=w371:errorcluster)  [unwired: 8 in, 1 out]
      }
      frame "SetStopOvl" {
        n180 = Unbundle By Name(w380) -> ("DevIdx"=w377:i32, "StopOvl."=w376:bool, "OvlLevel"=w375:u32)
        n181 = To Unsigned Long Integer(number=w375) -> (unsigned 32bit integer=w374:u32)
        n182 = call "MH_SetStopOverflow.vi"("stopcount"=w374, "StopOnOverflow"=w376, "devidx"=w377) -> ("error out"=w378:errorcluster)  [unwired: 7 in, 1 out]
      }
      frame "SetBitShift" {
        n183 = Unbundle By Name(w384) -> ("BitShift"=w382:i32, "SyncRate"=w383:i32)
        n184 = Negate(x=w382) -> (-x=w392:i32)
        n185 = Bundle By Name(cluster=T7 {"Cmd"=enum."Proc", "nActual"=0, "Buffer"=[], "TickCount"=0, "Param"=0} ("MH_DataProcThread_QData"), "Param"=w392, "Cmd"=MH_DataProcThread_QCmds."SetShift") -> (w398:T7)
        n186 = To Double Precision Float(number=w382) -> (double precision float=w397:dbl)
        n187 = To Double Precision Float(number=w383) -> (double precision float=w396:dbl)
        n188 = Power Of 2(x=w397) -> (2^x=w395:dbl)
        n189 = Enqueue Element(queue=w385, element=w398) -> ()  [unwired: 2 in, 3 out]
        n190 = Multiply(x=w395, y=1000.0) -> (x*y=w394:dbl)
        n191 = Divide(x=w394, y=w396) -> (x/y=w381:dbl)
        "DeltaT" <- w381
        n192 = Bundle By Name(cluster=T5 {"Histos"=[], "Cmd"=enum."_none_", "TimeTrace"=[], "Bin"=0, "Total bin"=0, "Status"="", "Resol"=0.0, "DeltaT"=0.0, "nChannels"=0} ("MH_GUIThread_QData"), "DeltaT"=w381, "Cmd"=MH_VisThread_QCmds."DeltaT") -> (w393:T5)
        n193 = Enqueue Element(queue=w386, element=w393) -> ()  [unwired: 2 in, 3 out]
      }
      frame "SetHistoAcqTime" {
        n194 = Unbundle By Name(w401) -> ("SyncRate"=w407:i32, "HistoAcqTime"=w400:dbl)
        n195 = To Double Precision Float(number=w407) -> (double precision float=w410:dbl)
        n196 = Multiply(x=w410, y=w400) -> (x*y=w409:dbl)
        n197 = Round To Nearest(number=w409) -> (nearest integer value=w408:dbl)
        n198 = To Long Integer(number=w408) -> (32bit integer=w406:i32)
        n199 = Bundle By Name(cluster=T7 {"Cmd"=enum."Proc", "nActual"=0, "Buffer"=[], "TickCount"=0, "Param"=0} ("MH_DataProcThread_QData"), "Param"=w406, "Cmd"=MH_DataProcThread_QCmds."SetHistAcqTime") -> (w405:T7)
        n200 = Enqueue Element(queue=w402, element=w405) -> ()  [unwired: 2 in, 3 out]
      }
      frame "GetAllRates" {
        # "An alternative to GetRates"
        n201 = Unbundle By Name(w415) -> ("DevIdx"=w417:i32, "Init Info.nchannels"=w420:i32)
        n202 = call "MH_AllocateCntRateBuffer.vi"("NumChan"=w420) -> ("Buffer"=w419:i32[])  [unwired: 10 in]
        n203 = call "MH_GetAllCountRates.vi"("cntrates_buf"=w419, "devidx"=w417) -> ("error out"=w414:errorcluster, "cntrates"=→"CountRates":i32[], "syncrate"=w418:i32)  [unwired: 6 in, 1 out]
        n204 = Format Into String(format string="Sync Rate: %d cps\n", w418) -> (resulting string=→"SyncRate":string)  [unwired: 2 in, 1 out]
      }
      frame "GetRates" {
        # "An alternative to GetAllRates"
        n205 = Unbundle By Name(w426) -> ("Init Info.nchannels"=w431:i32, "Channels"=w427:T2[], "DevIdx"=w428:i32)
        n206 = call "MH_GetSyncRate.vi"("devidx"=w428) -> ("error out"=w430:errorcluster, "syncrate"=w424:i32)  [unwired: 8 in, 1 out]
        n207 = Format Into String(format string="Sync Rate: %d cps\n", w424) -> (resulting string=w423:string)  [unwired: 2 in, 1 out]
        n208 = local write "SyncRate"(w423) -> ()
        n209 = for {
          N: w431 -> [_]
          tunnel: w428 -> [w439]
          tunnel: [w436] -> w422 mode=indexing
          shift-right: [w438] -> w432
          shift-left: w430 -> [w440]
          tunnel: w427 -> [w435] mode=indexing
          i -> [w437]
          n210 = Unbundle By Name(w435) -> ("Enable"=w434:bool)
          n211 = case shown="True" w434 {
            tunnel: w440 -> [w441 w446]
            tunnel: w439 -> [_ w445]
            tunnel: [w441 w444] -> w438
            tunnel: w437 -> [_ w443]
            tunnel: [_ w442] -> w436
            frame False {
            }
            frame True {
              n212 = call "MH_GetCountRate.vi"("error in (no error)"=w446, "Channel"=w443, "devidx"=w445) -> ("error out"=w444:errorcluster, "rate"=w442:i32)  [unwired: 6 in, 1 out]
            }
          }
        }
        n213 = local write "CountRates"(w422) -> ()
        n214 = Bundle By Name(cluster=w426, "SyncRate"=w424) -> (w425:T8)
      }
      frame "StartMeas" {
        n215 = Bundle By Name(cluster=T7 {"Cmd"=enum."Proc", "nActual"=0, "Buffer"=[], "TickCount"=0, "Param"=0} ("MH_DataProcThread_QData"), "Cmd"=MH_DataProcThread_QCmds."Init") -> (w448:T7)
        n216 = Unbundle By Name(w457) -> ("DevIdx"=w455:i32, "AcqTime"=w451:i32)
        n217 = Enqueue Element(queue=w450, element=w448) -> ()  [unwired: 2 in, 3 out]
        n218 = call "MH_StartMeas.vi"("tacq"=w451, "devidx"=w455) -> ("error out"=w456:errorcluster)  [unwired: 8 in, 1 out]
        n219 = Build Array (concatenate)(w454, MH_UIThread_Cmds."ReadFiFo") -> (w453:T10[])
      }
      frame "StopMeas" {
        n220 = Unbundle By Name(w463) -> ("Run cont."=w458:bool, "DevIdx"=w464:i32)
        n221 = call "MH_StopMeas.vi"("devidx"=w464) -> ("error out"=w465:errorcluster)  [unwired: 9 in, 1 out]
        n222 = case shown="True" w458 {
          tunnel: w463 -> [w469 w471]
          tunnel: [w468 w471] -> w462
          tunnel: [w466 w470] -> w461
          frame False {
            w466 = T10[] [enum."ReadFiFo"] items=["Idle", "Init", "SetInpChanEnable", "SetInpChanOffset", "SetInpChanTrg", "SetSyncDivider", "SetSyncTrg", "SetSyncOffset", "SetBinning", "SetHistoOffset", "SetHistoLen", "SetStopOvl", "SetBitShift", "SetHistoAcqTime", "GetRates", "GetAllRates", "StartMeas", "StopMeas", "AbortMeas", "GetResolution", "GetHistos", "GetAllHistos", "ReadFiFo", "WriteStatus", "Resize", "EnableControls", "DisableControls", "Error", "Exit"]
            w467 = FALSE ("StartMeas")
            n223 = Bundle By Name(cluster=w469, "StartMeas"=w467) -> (w468:T8)
            n224 = local write "Start"(w467) -> ()
          }
          frame True {
            w470 = T10[] [enum."ReadFiFo", enum."StartMeas"] items=["Idle", "Init", "SetInpChanEnable", "SetInpChanOffset", "SetInpChanTrg", "SetSyncDivider", "SetSyncTrg", "SetSyncOffset", "SetBinning", "SetHistoOffset", "SetHistoLen", "SetStopOvl", "SetBitShift", "SetHistoAcqTime", "GetRates", "GetAllRates", "StartMeas", "StopMeas", "AbortMeas", "GetResolution", "GetHistos", "GetAllHistos", "ReadFiFo", "WriteStatus", "Resize", "EnableControls", "DisableControls", "Error", "Exit"]
          }
        }
        n225 = Build Array (concatenate)(w460, w461) -> (w459:T10[])
      }
      frame "AbortMeas" {
        w473 = FALSE ("StartMeas")
        n226 = Unbundle By Name(w475) -> ("DevIdx"=w476:i32)
        n227 = call "MH_StopMeas.vi"("devidx"=w476) -> ("error out"=w477:errorcluster)  [unwired: 9 in, 1 out]
        n228 = Bundle By Name(cluster=w475, "StartMeas"=w473) -> (w474:T8)
        n229 = local write "Start"(w473) -> ()
      }
      frame "GetResolution" {
        # "Resolution in ns"
        # "Gets resolution in ps"
        # "Resolution is saved in UIThread Data cluster in ns"
        n230 = Unbundle By Name(w486) -> ("DevIdx"=w488:i32)
        n231 = call "MH_GetResolution.vi"("devidx"=w488) -> ("error out"=w487:errorcluster, "resolution"=w484:dbl)  [unwired: 8 in, 1 out]
        n232 = Divide(x=w484, y=1000.0) -> (x/y=w480:dbl)
        n233 = Bundle By Name(cluster=w486, "Resolution"=w480) -> (w485:T8)
        n234 = Bundle By Name(cluster=T5 {"Histos"=[], "Cmd"=enum."_none_", "TimeTrace"=[], "Bin"=0, "Total bin"=0, "Status"="", "Resol"=0.0, "DeltaT"=0.0, "nChannels"=0} ("MH_GUIThread_QData"), "Resol"=w480, "Cmd"=MH_VisThread_QCmds."Resol") -> (w478:T5)
        n235 = Enqueue Element(queue=w482, element=w478) -> ()  [unwired: 2 in, 3 out]
      }
      frame "ReadFiFo" {
        w498 = 2  # FLAG_FIFOFULL
        # "Reads photon records from HW and transferes them to DataProcThread via Queue."
        n236 = Unbundle By Name(w500) -> ("DevIdx"=w494:i32)
        n237 = call "MH_GetFlags.vi"("devidx"=w494) -> ("error out"=w496:errorcluster, "flags"=w497:i32)  [unwired: 8 in, 1 out]
        n238 = And(x=w497, y=w498) -> (x .and. y?=w499:i32)
        n239 = Not Equal To 0?(x=w499) -> (x != 0?=w493:bool)
        "OverRun" <- w493
        n240 = case shown="False" w493 {
          tunnel: w496 -> [w510 w513]
          tunnel: [w509 w513] -> w495
          tunnel: w494 -> [w502 _]
          tunnel: w492 -> [w508 _]
          tunnel: w491 -> [w507 _]
          tunnel: [w507 w511] -> w490
          frame False {
            n241 = call "MH_ReadFiFo.vi"("error in (no error)"=w510, "devidx"=w502) -> ("error out"=w509:errorcluster, "nactual"=w501:i32, "buffer"=w505:u32[])  [unwired: 6 in, 1 out]
            n242 = Bundle By Name(cluster=T7 {"Cmd"=enum."Proc", "nActual"=0, "Buffer"=[], "TickCount"=0, "Param"=0} ("MH_DataProcThread_QData"), "Buffer"=w505, "nActual"=w501, "Cmd"=MH_DataProcThread_QCmds."Proc") -> (w503:T7)
            n243 = Enqueue Element(queue=w508, element=w503) -> ()  [unwired: 2 in, 3 out]
          }
          frame True {
            n244 = Build Array(MH_UIThread_Cmds."AbortMeas") -> (w511:T10[])
          }
        }
      }
      frame "WriteStatus" {
        n245 = Unbundle By Name(w515) -> ("Status"=→"Status":string)
      }
      frame "Resize" {
        n246 = property on="Pane 3" class="Pane"() -> ("Width"=w522:u32)  [unwired: 2 in, 2 out]
        n247 = Subtract(x=w522, y=i16 100 ("b")) -> (x-y=w528:u32)
        n248 = Unbundle By Name(w517) -> ("Init Info.nchannels"=w525:i32)
        n249 = Quotient & Remainder(x=w528, y=i16 99 ("m")) -> (floor(x/y)=w527:u32)  [unwired: 1 out]
        n250 = In Range and Coerce(upper limit=w525, x=w527, lower limit=4) -> (coerced(x)=w526:u32)  [unwired: 1 out]
        n251 = Equal?(x=w525, y=w526) -> (x = y?=w524:bool)
        n252 = Not(x=w524) -> (.not. x?=w523:bool)
        n253 = property on="Channels" class="Arr (strict)"("HorizScroll"=w523, "Number of Columns"=w526, "Index Values"=u32[] [0]) -> ()  [unwired: 2 in, 2 out]
      }
      frame "EnableControls" {
        n254 = property class="VI"() -> ("Panel"=w533:refnum<vi>)  [unwired: 2 in, 2 out]
        n255 = property class="Pnl"(reference=w533) -> ("Controls[]"=w532:refnum<vi>[])  [unwired: 1 in, 2 out]
        n256 = property class="Pnl"(reference=w533) -> ("Decos[]"=w534:refnum<vi>[])  [unwired: 1 in, 2 out]
        n257 = for {
          tunnel: w534 -> [w538] mode=indexing
          tunnel: TRUE -> [w537]
          n258 = property class="Decor"(reference=w538, "Visible"=w537) -> ()  [unwired: 1 in, 2 out]
        }
        n259 = for {
          tunnel: w532 -> [w541] mode=indexing
          tunnel: T11."Enabled" ("Disabled") -> [w540]
          tunnel: [w539] -> _
          n260 = property class="Ctl"(reference=w541, "DisabledEnum"=w540) -> (error out=w539:errorcluster)  [unwired: 1 in, 1 out]
        }
      }
      frame "DisableControls" {
        n261 = property class="VI"() -> ("Panel"=w545:refnum<vi>)  [unwired: 2 in, 2 out]
        n262 = property class="Pnl"(reference=w545) -> ("Controls[]"=w544:refnum<vi>[])  [unwired: 1 in, 2 out]
        n263 = property class="Pnl"(reference=w545) -> ("Decos[]"=w546:refnum<vi>[])  [unwired: 1 in, 2 out]
        n264 = for {
          tunnel: w546 -> [w550] mode=indexing
          tunnel: FALSE -> [w549]
          n265 = property class="Decor"(reference=w550, "Visible"=w549) -> ()  [unwired: 1 in, 2 out]
        }
        n266 = for {
          tunnel: w544 -> [w553] mode=indexing
          tunnel: T11."Disabled and Grayed Out" ("Disabled") -> [w552]
          tunnel: [w551] -> _
          n267 = property class="Ctl"(reference=w553, "DisabledEnum"=w552) -> (error out=w551:errorcluster)  [unwired: 1 in, 1 out]
        }
      }
      frame "Error" {
        w554 = T10[] [enum."Exit"] items=["Idle", "Init", "SetInpChanEnable", "SetInpChanOffset", "SetInpChanTrg", "SetSyncDivider", "SetSyncTrg", "SetSyncOffset", "SetBinning", "SetHistoOffset", "SetHistoLen", "SetStopOvl", "SetBitShift", "SetHistoAcqTime", "GetRates", "GetAllRates", "StartMeas", "StopMeas", "AbortMeas", "GetResolution", "GetHistos", "GetAllHistos", "ReadFiFo", "WriteStatus", "Resize", "EnableControls", "DisableControls", "Error", "Exit"]
        w557 = T14 1 items=["no dialog", "OK message", "continue or stop message", "OK message + warnings", "continue/stop + warnings"] ("type of dialog (OK msg:1)")
        # "Error case: If an error occures the user is informed and the programm terminates. Add your own code to handle error events (e.g. exception lists, etc.)"
        n268 = call <vilib>:"Simple Error Handler.vi"("type of dialog (OK msg:1)"=w557, "error in (no error)"=w556) -> ()  [unwired: 3 in, 5 out]
      }
      frame "Exit" {
        n269 = Release Queue(queue=w559) -> ()  [unwired: 2 in, 3 out]
        n270 = Release Queue(queue=w558) -> ()  [unwired: 2 in, 3 out]
        n271 = Unbundle By Name(w563) -> ("DevIdx"=w562:i32)
        n272 = call "MH_CloseDevice.vi"("devidx"=w562) -> ("error out"=w561:errorcluster)  [unwired: 9 in, 1 out]
      }
    }
    n273 = call "MH_EnQError.vi"("error in (no error)"=w24, "Cmds_in"=w22) -> ("error out"=w23:errorcluster, "Cmds_out"=w21:T10[])  [unwired: 8 in]
  }
  n274 = call "MH_DataProcThread.vi"("MH_VisThread_QRef"=w7, "MH_DataProcThread_QRef"=w1) -> ()  [unwired: 10 in]
  n275 = while {
    tunnel: w7 -> [w572]
    shift-right: [w568] -> _
    shift-left: T4 {"Resol"=0.0, "DeltaT"=0.0, "NumChannels"=0} -> [w569]
    tunnel: w1 -> [w567]
    stop <- w565 stop-if-true
    # "VisualizationThread"
    n276 = Dequeue Element(queue=w572, timeout in ms (-1)=100) -> (element=w570:T5, error out=w565:errorcluster)  [unwired: 1 in, 2 out]
    n277 = Unbundle By Name(w570) -> ("Cmd"=w571:T6)
    n278 = case shown="\"Histo\"" w571 {
      tunnel: w570 -> [_ w585 w587 w599 w607 w611 w615]
      tunnel: w569 -> [w575 w583 w589 w591 w606 w610 w614]
      tunnel: [w575 w583 w588 w591 w606 w609 w613] -> w568
      tunnel: w567 -> [w574 _ _ _ w603 _ _]
      tunnel: w565 -> [w573 _ _ _ _ _ _]
      frame "_none_", Default {
        n279 = case shown="No Error" w573 {
          tunnel: w574 -> [w579 _]
          frame No Error {
            n280 = Get Queue Status(queue=w579) -> (# elements in queue=w577:i32)  [unwired: 2 in, 7 out]
            n281 = Format Into String(format string="Elements in Q: %d", w577) -> (resulting string=w576:string)  [unwired: 2 in, 1 out]
            n282 = local write "Status"(w576) -> ()
          }
          frame Error {
          }
        }
      }
      frame "Histo" {
        n283 = Unbundle By Name(w585) -> ("Histos"=w580:u32[][])
        n284 = Unbundle By Name(w583) -> ("Resol"=w582:dbl)
        n285 = Bundle(0.0, "Resol"=w582, "Histos"=w580) -> (→"HistoGraph":cluster{dbl, "Resol":dbl, "Histos":u32[][]})  [unwired: 1 in]
      }
      frame "nChannels" {
        n286 = Unbundle By Name(w587) -> ("nChannels"=w586:i32)
        n287 = Bundle By Name(cluster=w589, "NumChannels"=w586) -> (w588:T4)
      }
      frame "TTrace" {
        n288 = Unbundle By Name(w599) -> ("Total bin"=w598:u64, "Bin"=w597:i32, "TimeTrace"=w596:u32[][])
        n289 = Unbundle By Name(w591) -> ("DeltaT"=w590:dbl)
        n290 = call "MH_TTraceToGraph.vi"("DeltaT"=w590, "TimeTrace"=w596, "Bin"=w597, "Total bin"=w598) -> ("TimeTrace_out"=w593:u32[][], "dt"=w594:dbl, "T0"=w595:dbl)  [unwired: 5 in]
        n291 = Bundle("T0"=w595, "dt"=w594, "TimeTrace_out"=w593) -> (→"TTraceGraph":T15)  [unwired: 1 in]
      }
      frame "Status" {
        n292 = Unbundle By Name(w607) -> ("Status"=w604:string)
        n293 = Get Queue Status(queue=w603) -> (# elements in queue=w602:i32)  [unwired: 2 in, 7 out]
        n294 = Format Into String(format string="\t\tElements in Q: %d", w602) -> (resulting string=w600:string)  [unwired: 2 in, 1 out]
        n295 = Concatenate Strings(w604, w600) -> (w605:string)
        n296 = local write "Status"(w605) -> ()
      }
      frame "DeltaT" {
        n297 = Unbundle By Name(w611) -> ("DeltaT"=w608:dbl)
        n298 = Bundle By Name(cluster=w610, "DeltaT"=w608) -> (w609:T4)
      }
      frame "Resol" {
        n299 = Unbundle By Name(w615) -> ("Resol"=w612:dbl)
        n300 = Bundle By Name(cluster=w614, "Resol"=w612) -> (w613:T4)
      }
    }
  }
